vi "LogStartTimeGlobal.vi"(7 "Action":T1, 11 "Set Value":timestamp) -> (3 "Value Out":timestamp)   [LabVIEW 2013]
uses:
  LogStartTimeGlobalAction.ctl
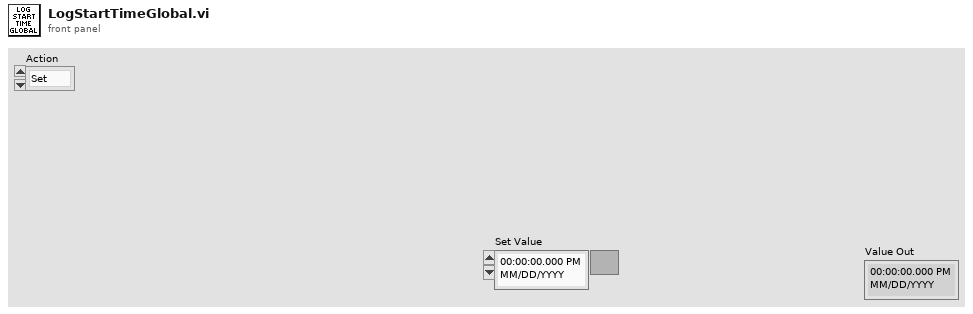
[diagram p1: front panel]
types:
  T1 = typedef "LogStartTimeGlobalAction.ctl" = enum16{"Set", "Get"}
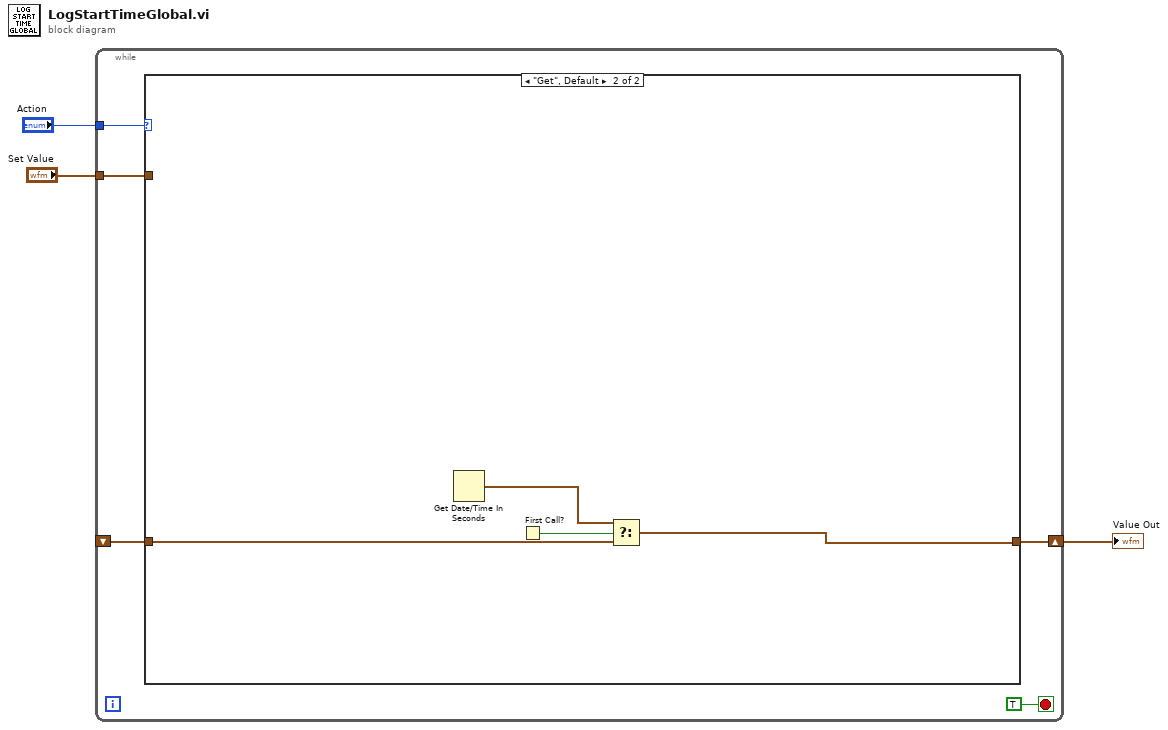
[diagram p0: block diagram]
diagram:
  n1 = while {
    tunnel: "Action" -> [w7]
    tunnel: "Set Value" -> [w6]
    shift-right: [w5] -> w1
    shift-left: _ -> [w4]
    stop <- TRUE stop-if-true
    n2 = case shown="\"Get\", Default" w7 {
      tunnel: w6 -> [w9 _]
      tunnel: [w9 w12] -> w5
      tunnel: w4 -> [_ w11]
      frame "Set" {
      }
      frame "Get", Default {
        n3 = Get Date/Time In Seconds() -> (seconds since 1Jan1904=w10:timestamp)
        n4 = First Call?() -> (First Call?: T/F=w13:bool)
        n5 = Select(t=w10, s=w13, f=w11) -> (s? t:f=w12:timestamp)
      }
    }
  }
  "Value Out" <- w1
